vi "Configure Security.vi"(0 "VISA resource name":refnum<visa-resource-name>, 7 "Security On/OFF (F:Off)":bool, 11 "error in (no error)":errorcluster) -> (4 "VISA resource name out":refnum<visa-resource-name>, 15 "error out":errorcluster)   [LabVIEW 2020, in "eec EST 300.lvlib"]
doc: "SL {1|0}\nSets the Security function ON or OFF\n\nOFF: Disable security features\nON: Programmable User ID and Password capability to avoid unauthorized access to test set-up program."
uses:
  <instrlib>/eec EST 300/eec EST 300.lvlib
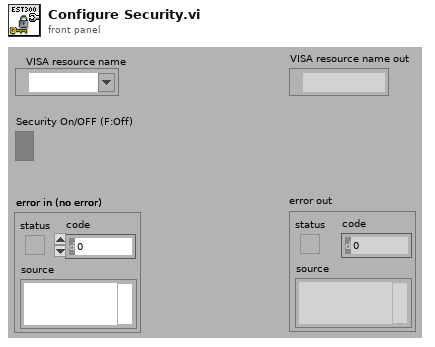
[diagram p1: front panel]
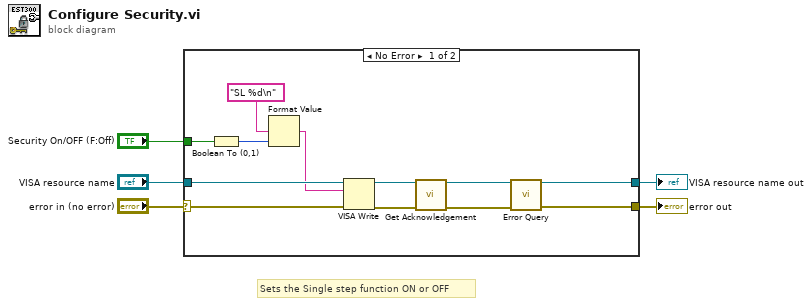
[diagram p0: block diagram]
diagram:
  # "Sets the Single step function ON or OFF"
  n1 = case shown="No Error" "error in (no error)" {
    selector: "error in (no error)" -> [w16 w19]
    tunnel: [w7 w19] -> w4
    tunnel: [w8 w18] -> w2
    tunnel: "VISA resource name" -> [w17 w18]
    tunnel: "Security On/OFF (F:Off)" -> [w15 _]
    frame No Error {
      n2 = Boolean To (0,1)(Boolean=w15) -> (0, 1=w6:i16)
      n3 = Format Value(format string="SL %d\n", value (0)=w6) -> (output string=w13:string)  [unwired: 1 in]
      n4 = VISA Write(VISA resource name=w17, write buffer=w13, error in (no error)=w16) -> (VISA resource name out=w10:refnum<visa-resource-name>, error out=w9:errorcluster)  [unwired: 1 out]
      n5 = call <instrlib>:"Get Acknowledgement.vi"("VISA resource name"=w10, "error in (no error)"=w9) -> ("VISA resource name out"=w12:refnum<visa-resource-name>, "error out"=w11:errorcluster)  [unwired: 12 in]
      n6 = call <instrlib>:"Error Query.vi"("VISA resource name"=w12, "error in (no error)"=w11) -> ("VISA resource name out"=w8:refnum<visa-resource-name>, "error out"=w7:errorcluster)  [unwired: 10 in, 2 out]
    }
    frame Error {
    }
  }
  "error out" <- w4
  "VISA resource name out" <- w2
